vi "SHIFT_HIGH.vi"(10 "argv":string[](array[string]), 11 "args":u8) -> ()   [LabVIEW 2014]
uses:
  TORC Code/GlobalVariable.vi
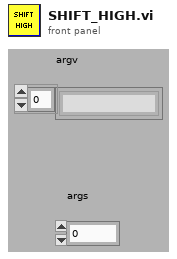
[diagram p1: front panel]
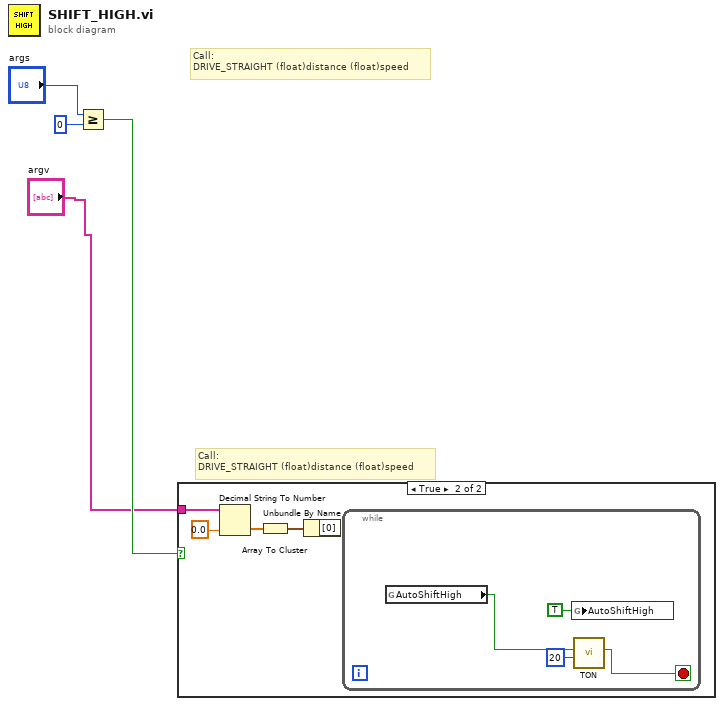
[diagram p0: block diagram]
diagram:
  # "Call:\nDRIVE_STRAIGHT (float)distance (float)speed"
  # "Call:\nDRIVE_STRAIGHT (float)distance (float)speed"
  n1 = Greater Or Equal?(x="args", y=u8 0) -> (x >= y?=w4:bool)
  n2 = case shown="True" w4 {
    tunnel: "argv" -> [_ w8]
    frame False {
    }
    frame True {
      n3 = Decimal String To Number(string=w8, default (0L)=0.0 ("default (0 I32)")) -> (number=w6:dbl[])  [unwired: 2 out]
      n4 = Array To Cluster(array=w6) -> (cluster=w5:cluster{"[0]":dbl, "[1]":dbl})
      n5 = Unbundle By Name(w5) -> ()  [unwired: 1 out]
      n6 = while {
        stop <- w9 stop-if-true
        n7 = global read "GlobalVariable.vi" "AutoShiftHigh"() -> (w11:bool)
        n8 = global write "GlobalVariable.vi" "AutoShiftHigh"(TRUE ("AutoShiftHigh")) -> ()
        n9 = call "TON.vi"("Delay (ms)"=u32 20 ("Delay ms"), "Input"=w11) -> ("Output"=w9:bool)  [unwired: 9 in]
      }
    }
  }
